vi "Create Today's Page.vi"(10 "User Email":string="myemail", 11 "Notebook Name":string="My notebook on One Drive") -> (0 "error out":errorcluster, 3 "headers":string)   [LabVIEW 2019, in "OneNote Library.lvlib"]
uses:
  OneNote Library.lvlib
  <vilib>/httpClient/POSTBuffer.vi
  <vilib>/httpClient/LabVIEWHTTPClient.lvlib
panel:
  out "body":string
  out "Result":string
  out "date/time string":string
  out "LabVIEW TimeStamp":timestamp
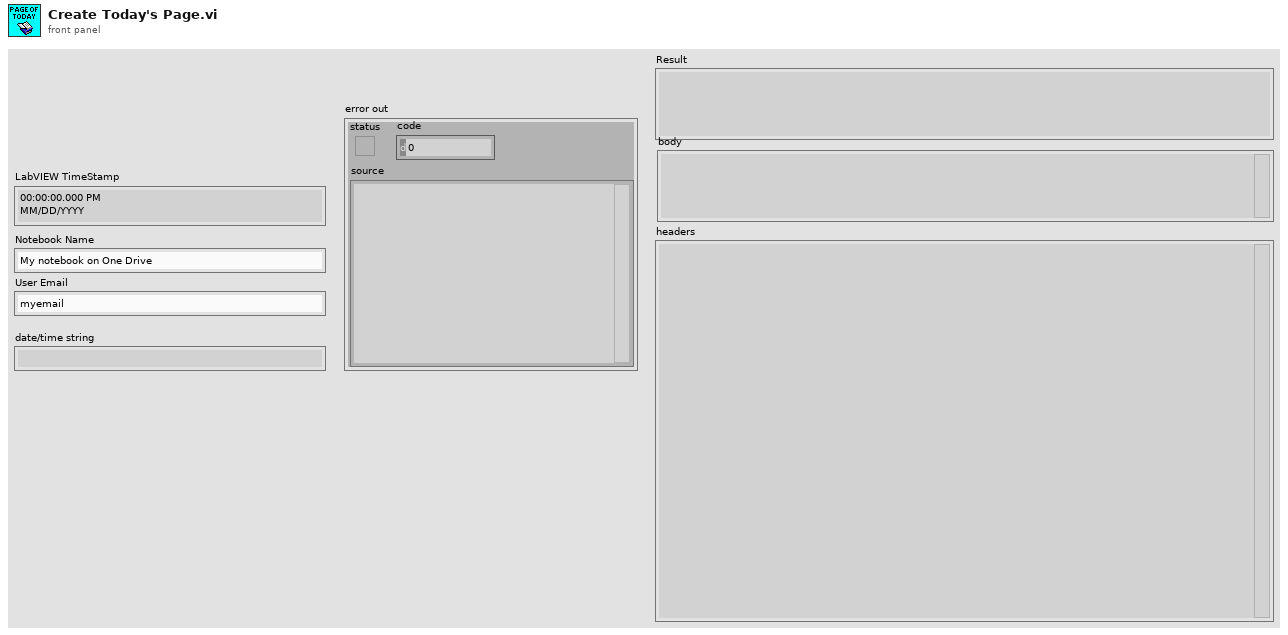
[diagram p1: front panel]
types:
  T1 = typedef "LabVIEWHTTPClient.lvlib/ClientHandle.ctl" = refnum<k1>
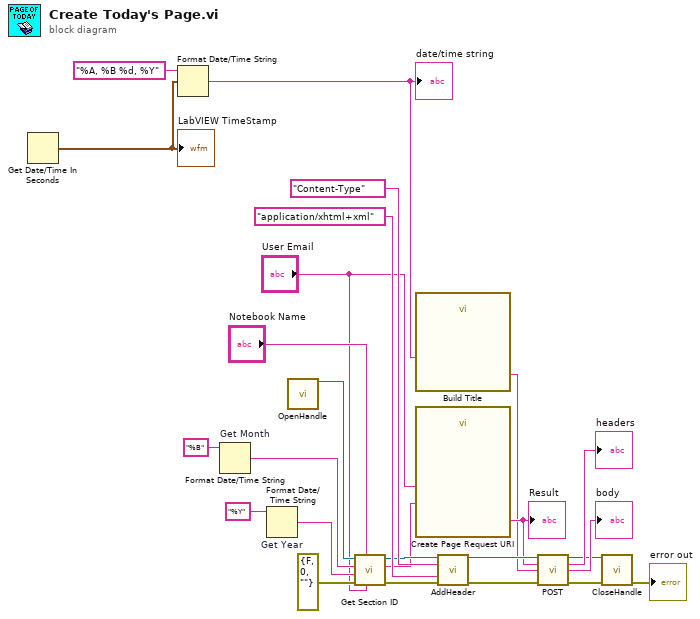
[diagram p0: block diagram]
diagram:
  n1 = Get Date/Time In Seconds() -> (seconds since 1Jan1904=w25:timestamp)
  "LabVIEW TimeStamp" <- w25
  n2 = Format Date/Time String(time format string (%c)="%A, %B %d, %Y", seconds (now)=w25) -> (date/time string=w7:string)  [unwired: 1 in]
  "date/time string" <- w7
  n3 = Format Date/Time String "Get Month"(time format string (%c)="%B") -> (date/time string=w21:string)  [unwired: 2 in]
  n4 = Format Date/Time String "Get Year"(time format string (%c)="%Y") -> (date/time string=w20:string)  [unwired: 2 in]
  n5 = call <vilib>:"OpenHandle.vi"() -> ("client handle out"=w17:T1)  [unwired: 14 in, 1 out]
  n6 = call "Get Section ID.vi"("User Email"="User Email", "Notebook Name"="Notebook Name", "Error In (No Error)"=errorcluster {"status"=FALSE, "code"=0, "source"=""}, "Year (Section Group)"=w20, "Month (Section)"=w21, "client handle"=w17) -> ("error out"=w14:errorcluster, "Section ID"=w9:string, "client handle out"=w12:T1)  [unwired: 3 in]
  n7 = call "Build Title"("Title"=w7) -> ("Result"=w6:string)  [unwired: 13 in, 1 out]
  n8 = call "Create Page Request URI"("user email"="User Email", "Section ID"=w9) -> ("Result"=w8:string)  [unwired: 12 in, 1 out]
  "Result" <- w8
  n9 = call <vilib>:"AddHeader.vi"("client handle"=w12, "header"="Content-Type", "value"="application/xhtml+xml", "error in (no error)"=w14) -> ("client handle out"=w13:T1, "error out"=w11:errorcluster)  [unwired: 10 in]
  n10 = call-poly <vilib>:"POST.vi"("client handle"=w13, "url"=w8, "buffer"=w6, "error in (no error)"=w11) -> ("client handle out"=w3:T1, "headers"=→"headers":string, "body"=→"body":string, "error out"=w2:errorcluster)  [unwired: 8 in]
  n11 = call <vilib>:"CloseHandle.vi"("client handle"=w3, "error in (no error)"=w2) -> ("error out"=→"error out":errorcluster)  [unwired: 13 in]
